vi "Set Angle Limits.vi"(8 "error in (no error)":errorcluster, 9 "min angle (rad)":dbl, 10 "max angle (rad)":dbl, 11 "KUKA youBot arm motor in":refnum<class "NI_Robotics_KUKA youBot Arm Motor.lvclass">) -> (0 "error out":errorcluster, 3 "KUKA youBot arm motor out":refnum<class "NI_Robotics_KUKA youBot Arm Motor.lvclass">)   [LabVIEW 2017, in "NI_Robotics_KUKA youBot Host.lvlib" / "NI_Robotics_KUKA youBot Arm Motor.lvclass"]
uses:
  <vilib>/robotics/KUKA youBot/Motor/Arm Motor/NI_Robotics_KUKA youBot Arm Motor.lvclass
  <vilib>/robotics/KUKA youBot/Motor/Arm Motor/NI_Robotics_KUKA youBot Arm Motor.lvclass/NI_Robotics_KUKA youBot Arm Motor.ctl
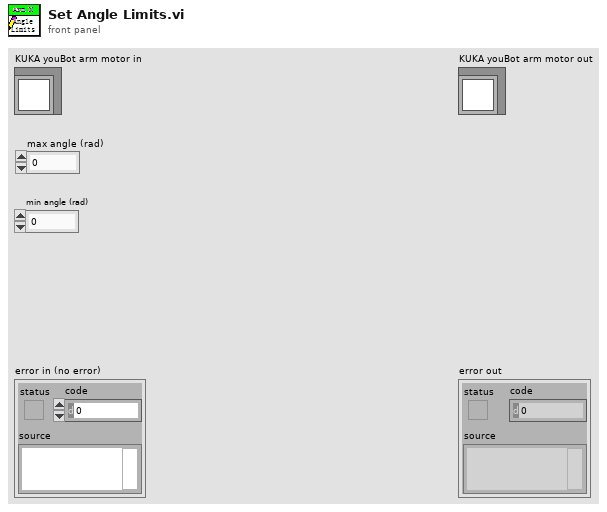
[diagram p1: front panel]
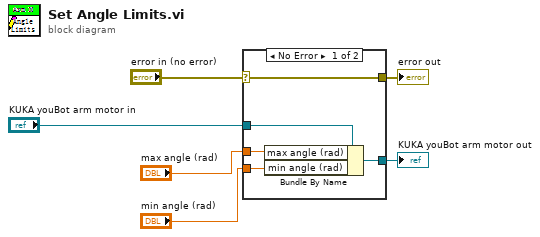
[diagram p0: block diagram]
diagram:
  n1 = case shown="No Error" "error in (no error)" {
    selector: "error in (no error)" -> [w11 w12]
    tunnel: [w11 w12] -> w5
    tunnel: [w9 w13] -> w3
    tunnel: "KUKA youBot arm motor in" -> [w10 w13]
    tunnel: "min angle (rad)" -> [w8 _]
    tunnel: "max angle (rad)" -> [w7 _]
    frame No Error {
      n2 = Bundle By Name(cluster=w10, "max angle (rad)"=w7, "min angle (rad)"=w8) -> (w9:refnum<class "NI_Robotics_KUKA youBot Arm Motor.lvclass">)
    }
    frame Error {
    }
  }
  "error out" <- w5
  "KUKA youBot arm motor out" <- w3
